vi "addPixmap.vi"(6 "state (Off)":T1=1 items=["On", "Off"], 8 "Error In":errorcluster, 9 "mode (Normal)":T2 items=["Normal", "Disabled", "Active", "Selected"], 10 "pixmap":refnum<class "QPixmap.lvclass">, 11 "QIcon In":refnum<class "QIcon.lvclass">) -> (0 "Error Out":errorcluster, 3 "QIcon Out":refnum<class "QIcon.lvclass">)   [LabVIEW 2014, in "QIcon.lvclass"]
doc: "LabVIEW-specific documentation is not yet available. See <b>https://doc.qt.io/qt-5/qicon.html#addPixmap</b>"
uses:
  QIcon.lvclass
  QPixmap/QPixmap.lvclass
  Mode.ctl
  State.ctl
  LQ Core/LQSerialData/LQSerialData.lvclass/LQSerialData.ctl
  LQ Core/LQ Core.lvlib
  LQ Core/LQSerialData/LQSerialData.lvclass
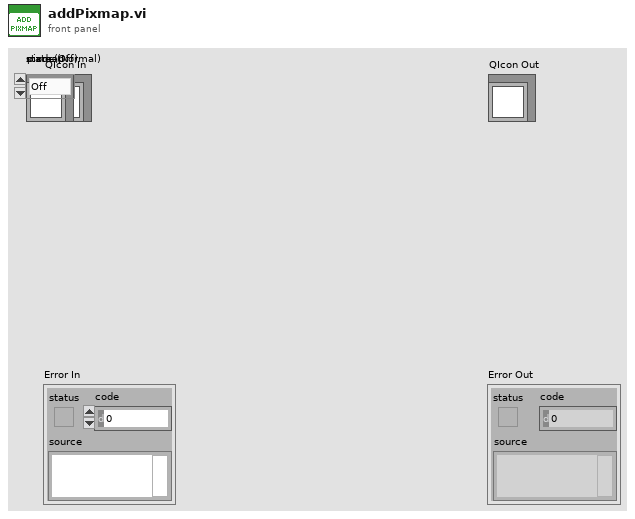
[diagram p1: front panel]
types:
  T1 = typedef "QIcon.lvclass/State.ctl" = i32
  T2 = typedef "QIcon.lvclass/Mode.ctl" = i32
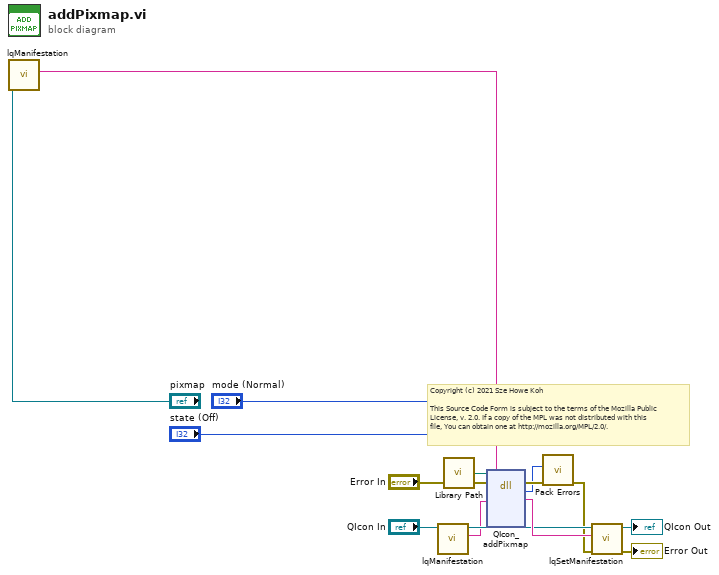
[diagram p0: block diagram]
diagram:
  # "Copyright (c) 2021 Sze Howe Koh\n\nThis Source Code Form is subject to the terms of the Mozilla Public\nLicense, v. 2.0. If a copy of the MPL was not distributed with this\nfile, You can obtain one at http://mozilla.org/MPL/2.0/."
  n1 = call "lqManifestation.vi"("LQSerialData in"="pixmap") -> ("Manifestation"=w3:string)  [unwired: 9 in, 1 out]
  n2 = call "lqManifestation.vi"("LQSerialData in"="QIcon In") -> ("Manifestation"=w10:string, "LQSerialData out"=w11:refnum<class "QIcon.lvclass">)  [unwired: 9 in]
  n3 = call "Library Path.vi"() -> ("Library Path"=w9:path)
  n4 = dll-call lib="?" fn="QIcon_addPixmap"(path in=w9, error in="Error In", "_instance"=w10, "pixmap"=w3, "mode"="mode (Normal)", "state"="state (Off)") -> (error out=w8:errorcluster, w7:i32, "_instance"=w13:string)  [unwired: 4 in, 1 out]
  n5 = call "Pack Errors.vi"("Error In"=w8, "Error Code"=w7) -> ("Error Out"=w6:errorcluster)  [unwired: 9 in]
  n6 = call "lqSetManifestation.vi"("Error In"=w6, "Manifestation"=w13, "LQSerialData in"=w11) -> ("Error Out"=→"Error Out":errorcluster, "LQSerialData out"=→"QIcon Out":refnum<class "QIcon.lvclass">)  [unwired: 7 in]
